vi "Main.vi"() -> ()   [LabVIEW 2019]
uses:
  <vilib>/sound2/lvsound2.llb/Sound Data Format.ctl
  <vilib>/sound2/lvsound2.llb/Sampling Mode.ctl
  <vilib>/sound2/lvsound2.llb/Sound Input Read (DBL).vi
panel:
  out "Raw Data":waveform(dbl)[](graph)
  out "error out":errorcluster
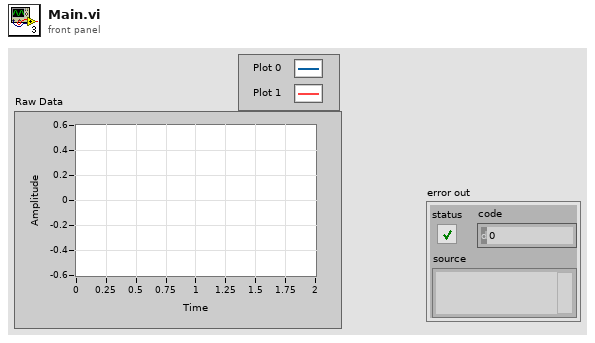
[diagram p1: front panel]
types:
  T1 = typedef "Sampling Mode.ctl" = i32
  T2 = typedef "Sound Data Format.ctl" = cluster{"sample rate (S/s)":dbl, "number of channels":i32, "bits per sample":i32}
  T3 = typedef "Sound Input Task ID.ctl" = u32
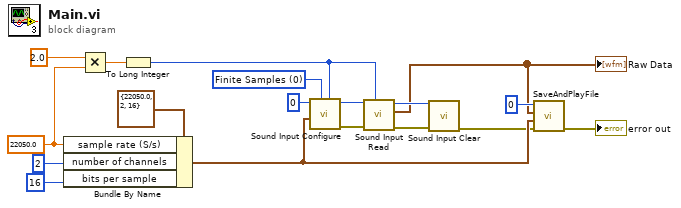
[diagram p0: block diagram]
diagram:
  w10 = T1 0 items=["Finite Samples", "Continuous Samples"] ("sample mode")
  w4 = 22050.0 ("Sample rate (Hz)")
  n1 = Bundle By Name(cluster=T2 {"sample rate (S/s)"=22050.0, "number of channels"=2, "bits per sample"=16} ("Sound Format"), "sample rate (S/s)"=w4, "number of channels"=2 ("#Channels"), "bits per sample"=16 ("Resolution (bits)")) -> (w3:T2)
  n2 = Multiply(x=2.0 ("Duration (s)"), y=w4) -> (x*y=w8:dbl)
  n3 = To Long Integer(number=w8) -> (32bit integer=w7:i32)
  n4 = call <vilib>:"Sound Input Configure.vi"("number of samples/ch"=w7, "sample mode"=w10, "sound format"=w3, "device ID"=u32 0 ("Device")) -> ("error out"=w13:errorcluster, "task ID"=w9:T3)  [unwired: 6 in]
  n5 = call-poly <vilib>:"Sound Input Read.vi"("number of samples/ch"=w7, "error in (no error)"=w13, "task ID"=w9) -> ("error out"=w5:errorcluster, "data"=w1:waveform(dbl)[], "task ID out"=w6:T3)  [unwired: 6 in]
  "Raw Data" <- w1
  n6 = call <vilib>:"Sound Input Clear.vi"("error in (no error)"=w5, "task ID"=w6) -> ("error out"=w2:errorcluster)  [unwired: 9 in]
  n7 = call "SaveAndPlayFile.vi"("error in (no error)"=w2, "Sound Format"=w3, "Waveform(s) in"=w1, "Speaker device ID"=u32 0 ("Device")) -> ("error out"=→"error out":errorcluster)  [unwired: 7 in]
